vi "Run Tests in Active Project.vi"(10 "Virtual Folder (empty: \"My Computer\")":string) -> ()   [LabVIEW 2013]
uses:
  classes/Test Runner/Test Runner.lvclass/Test Runner.ctl
  classes/Test Runner.Project/Test Runner.Project.lvclass
  classes/Test Runner/Test Runner.lvclass
panel:
  out "error out":errorcluster
  # "CARAYA Run Active Project's Unit Tests\n\nThis tool will run all Caraya Unit Tests found in the active project."
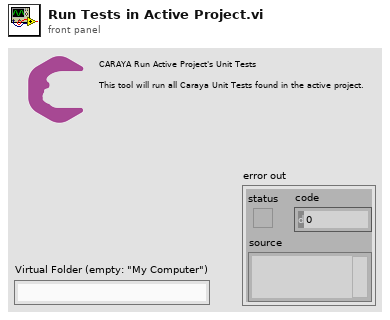
[diagram p1: front panel]
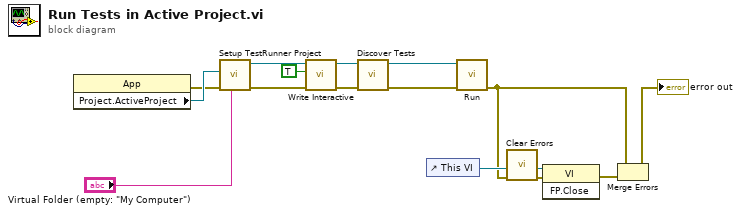
[diagram p0: block diagram]
diagram:
  n1 = property on="Property Node" class="App"() -> (error out=w12:errorcluster, "Project.ActiveProject"=w14:refnum<vi>)  [unwired: 2 in, 1 out]
  n2 = call "Setup TestRunner Project.vi"("Virtual Folder (empty: \"My Computer\")"="Virtual Folder (empty: \"My Computer\")", "error in (no error)"=w12, "Project Refnum"=w14) -> ("error out"=w13:errorcluster, "Test Runner.Project out"=w10:refnum<class "Test Runner.Project.lvclass">)  [unwired: 7 in]
  n3 = call "Write Interactive.vi"("Interactive"=TRUE, "Test Runner in"=w10) -> ("Test Runner out"=w9:refnum<class "Test Runner.Project.lvclass">)  [unwired: 9 in]
  n4 = call "Discover Tests.vi"("error in (no error)"=w13, "Test Runner in"=w9) -> ("error out"=w6:errorcluster, "Test Runner out"=w7:refnum<class "Test Runner.Project.lvclass">)  [unwired: 8 in]
  n5 = control-ref of="This VI"() -> (w5:refnum<vi>)
  n6 = call "Run.vi"("error in (no error)"=w6, "Test Runner in"=w7) -> ("error out"=w2:errorcluster)  [unwired: 8 in, 1 out]
  n7 = call <vilib>:"Clear Errors.vi"("error in (no error)"=w2) -> ("error out"=w1:errorcluster)  [unwired: 6 in]
  n8 = invoke class="VI" method="FP.Close"(reference=w5, error in=w1) -> (error out=w4:errorcluster)  [unwired: 1 in, 2 out]
  n9 = Merge Errors(w2, w4) -> (→"error out":errorcluster)
